vi "Parse GSA Sentence.vi"(8 "error in (no error)":errorcluster, 11 "GSA sentence":string) -> (0 "error out":errorcluster, 3 "GSA data":T1 {"type of fix"."mode" items=["", "No Fix", "2D Fix", "3D Fix"]; "selection of fix"."selection of 2D or 3D fix" items=["Automatic", "Manual"]})   [LabVIEW 2017, in "NMEA API.lvlib"]
doc: "Returns data contained in a particular type of NMEA sentence. The input sentence you specify must include valid NMEA formatting and end with a carriage return and line feed, or \\r\\n. You must manually select the polymorphic instance to use."
uses:
  <vilib>/robotics/Protocols/NMEA/NMEA API.lvlib
  <vilib>/robotics/Protocols/NMEA/typedefs/GSA Data.ctl
  <vilib>/robotics/Utilities/NI_Robotics Utilities.lvlib
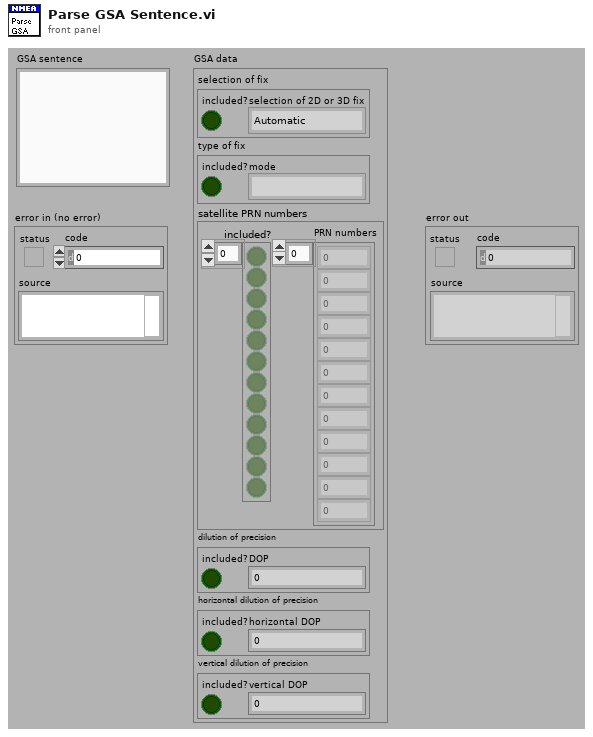
[diagram p1: front panel]
types:
  T1 = typedef "NMEA API.lvlib/GSA Data.ctl" = cluster{"selection of fix":cluster{"included?":bool, "selection of 2D or 3D fix":u16}, "type of fix":cluster{"included?":bool, "mode":u16}, "satellite PRN numbers":cluster{"included?":bool[], "PRN numbers":i32[]}, "dilution of precision":cluster{"included?":bool, "DOP":dbl}, "horizontal dilution of precision":cluster{"included?":bool, "horizontal DOP":dbl}, "vertical dilution of precision":cluster{"included?":bool, "vertical DOP":dbl}}
  T2 = cluster{"Included?":bool[], "Satellite PRNs":i32[]}
  T3 = cluster{"Valid?":bool, "Selection of 2D or 3D Fix":u16}
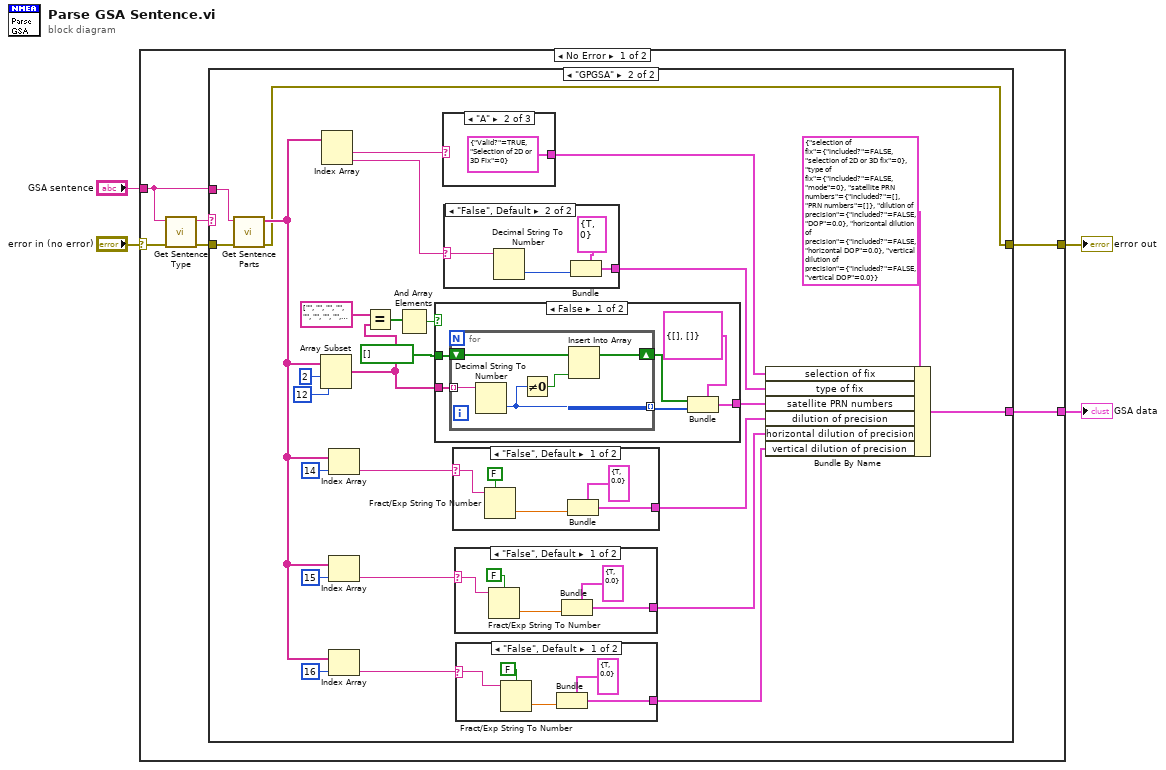
[diagram p0: block diagram]
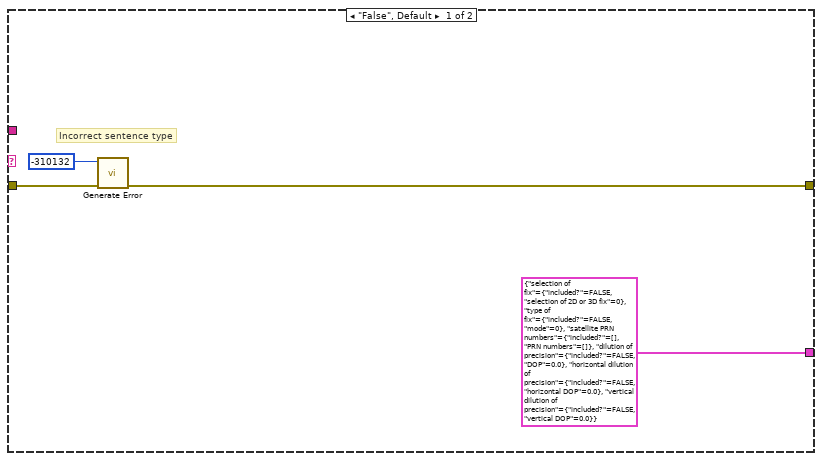
[diagram p2: hidden frame]
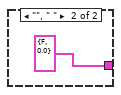
[diagram p3: hidden frame]
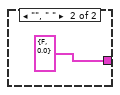
[diagram p4: hidden frame]
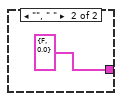
[diagram p5: hidden frame]
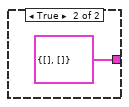
[diagram p6: hidden frame]
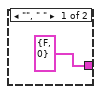
[diagram p7: hidden frame]
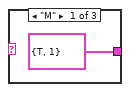
[diagram p8: hidden frame]
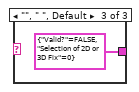
[diagram p9: hidden frame]
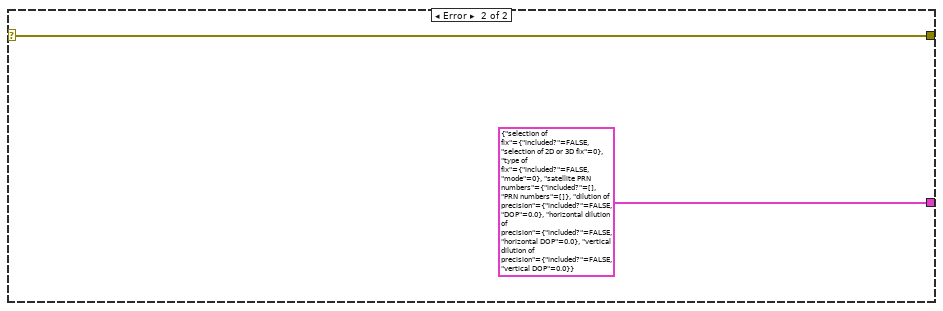
[diagram p10: hidden frame]
diagram:
  n1 = case shown="No Error" "error in (no error)" {
    selector: "error in (no error)" -> [w8 w81]
    tunnel: [w9 w81] -> w2
    tunnel: [w10 T1 {"selection of fix"={"included?"=FALSE, "selection of 2D or 3D fix"=0}, "type of fix"={"included?"=FALSE, "mode"=0}, "satellite PRN numbers"={"included?"=[], "PRN numbers"=[]}, "dilution of precision"={"included?"=FALSE, "DOP"=0.0}, "horizontal dilution of precision"={"included?"=FALSE, "horizontal DOP"=0.0}, "vertical dilution of precision"={"included?"=FALSE, "vertical DOP"=0.0}} ("GSA Data")] -> w1
    tunnel: "GSA sentence" -> [w6 _]
    frame No Error {
      n2 = call <vilib>:"Get Sentence Type.vi"("error in (no error)"=w8, "sentence"=w6) -> ("error out"=w7:errorcluster, "sentence type"=w5:string)  [unwired: 1 in, 7 out]
      n3 = case shown="\"GPGSA\"" w5 {
        tunnel: w6 -> [_ w16]
        tunnel: w7 -> [w12 w41]
        tunnel: [T1 {"selection of fix"={"included?"=FALSE, "selection of 2D or 3D fix"=0}, "type of fix"={"included?"=FALSE, "mode"=0}, "satellite PRN numbers"={"included?"=[], "PRN numbers"=[]}, "dilution of precision"={"included?"=FALSE, "DOP"=0.0}, "horizontal dilution of precision"={"included?"=FALSE, "horizontal DOP"=0.0}, "vertical dilution of precision"={"included?"=FALSE, "vertical DOP"=0.0}} ("GSA Data") w20] -> w10
        tunnel: [w11 w15] -> w9
        frame "False", Default {
          # "Incorrect sentence type"
          n4 = call <vilib>:"Generate Error.vi"("error in (no error)"=w12, "code"=-310132) -> ("error out"=w11:errorcluster)  [unwired: 9 in]
        }
        frame "GPGSA" {
          n5 = call <vilib>:"Get Sentence Parts.vi"("error in (no error)"=w41, "sentence"=w16) -> ("error out"=w15:errorcluster, "sentence data"=w17:string[])  [unwired: 1 in, 7 out]
          n6 = Array Subset(array=w17, index=2, length=12) -> (w32:string[])
          n7 = Index Array(array=w17) -> (element #1=w40:string, element #2=w36:string)  [unwired: 2 in]
          n8 = Index Array(array=w17, index=14) -> (element=w27:string)
          n9 = Index Array(array=w17, index=15) -> (element=w25:string)
          n10 = Index Array(array=w17, index=16) -> (element=w23:string)
          n11 = Equal?(x=string[] ["", "", "", "", "", "", "", "", "", "", "", ""], y=w32) -> (x = y?=w30:bool[])
          n12 = And Array Elements(Boolean array=w30) -> (logical AND=w29:bool)
          n13 = case shown="False" w29 {
            tunnel: w32 -> [w65 _]
            tunnel: [w62 T2 {"Included?"=[], "Satellite PRNs"=[]} ("Satellite PRNs")] -> w19
            tunnel: bool[] [] ("Included?") -> [w61 _]
            frame False {
              n14 = for {
                tunnel: [w66] -> w64 mode=indexing
                tunnel: w65 -> [w70] mode=indexing
                shift-right: [w68] -> w60
                shift-left: w61 -> [w69]
                n15 = Decimal String To Number(string=w70) -> (number=w66:i32)  [unwired: 3 out]
                n16 = Not Equal To 0?(x=w66) -> (x != 0?=w67:bool)
                n17 = Insert Into Array(array=w69, new element=w67) -> (w68:bool[])  [unwired: 1 in]
              }
              n18 = Bundle(cluster=T2 {"Included?"=[], "Satellite PRNs"=[]} ("Satellite PRNs"), "Included?"=w60, "Satellite PRNs"=w64) -> (w62:T2)
            }
            frame True {
            }
          }
          n19 = case shown="\"A\"" w40 {
            tunnel: [T3 {"Valid?"=TRUE, "Selection of 2D or 3D Fix"=1} ("Selection of Fix") T3 {"Valid?"=TRUE, "Selection of 2D or 3D Fix"=0} ("Selection of Fix") T3 {"Valid?"=FALSE, "Selection of 2D or 3D Fix"=0} ("Selection of Fix")] -> w35
            frame "M" {
            }
            frame "A" {
            }
            frame "", " ", Default {
            }
          }
          n20 = case shown="\"False\", Default" w36 {
            selector: w36 -> [_ w76]
            tunnel: [cluster{"Valid?":bool, "Type of Fix":u16} {"Valid?"=FALSE, "Type of Fix"=0} ("Type of Fix") w73] -> w28
            frame "", " " {
            }
            frame "False", Default {
              n21 = Decimal String To Number(string=w76) -> (number=w74:i32)  [unwired: 3 out]
              n22 = Bundle(cluster=cluster{"Valid?":bool, "Type of Fix":u16} {"Valid?"=TRUE, "Type of Fix"=0} ("Type of Fix"), "Type of Fix"=w74) -> (w73:cluster{"Valid?":bool, "Type of Fix":u16})  [unwired: 1 out]
            }
          }
          n23 = case shown="\"False\", Default" w27 {
            selector: w27 -> [w58 _]
            tunnel: [w55 cluster{"Valid?":bool, "DOP":dbl} {"Valid?"=FALSE, "DOP"=0.0} ("Dilution of Precision")] -> w26
            frame "False", Default {
              n24 = Fract/Exp String To Number(use system decimal point (T)=FALSE, string=w58) -> (number=w56:dbl)  [unwired: 3 out]
              n25 = Bundle(cluster=cluster{"Valid?":bool, "DOP":dbl} {"Valid?"=TRUE, "DOP"=0.0} ("Dilution of Precision"), "DOP"=w56) -> (w55:cluster{"Valid?":bool, "DOP":dbl})  [unwired: 1 out]
            }
            frame "", " " {
            }
          }
          n26 = case shown="\"False\", Default" w25 {
            selector: w25 -> [w52 _]
            tunnel: [w49 cluster{"Valid?":bool, "DOP":dbl} {"Valid?"=FALSE, "DOP"=0.0} ("Dilution of Precision")] -> w24
            frame "False", Default {
              n27 = Fract/Exp String To Number(use system decimal point (T)=FALSE, string=w52) -> (number=w50:dbl)  [unwired: 3 out]
              n28 = Bundle(cluster=cluster{"Valid?":bool, "DOP":dbl} {"Valid?"=TRUE, "DOP"=0.0} ("Dilution of Precision"), "DOP"=w50) -> (w49:cluster{"Valid?":bool, "DOP":dbl})  [unwired: 1 out]
            }
            frame "", " " {
            }
          }
          n29 = case shown="\"False\", Default" w23 {
            selector: w23 -> [w46 _]
            tunnel: [w43 cluster{"Valid?":bool, "DOP":dbl} {"Valid?"=FALSE, "DOP"=0.0} ("Dilution of Precision")] -> w22
            frame "False", Default {
              n30 = Fract/Exp String To Number(use system decimal point (T)=FALSE, string=w46) -> (number=w44:dbl)  [unwired: 3 out]
              n31 = Bundle(cluster=cluster{"Valid?":bool, "DOP":dbl} {"Valid?"=TRUE, "DOP"=0.0} ("Dilution of Precision"), "DOP"=w44) -> (w43:cluster{"Valid?":bool, "DOP":dbl})  [unwired: 1 out]
            }
            frame "", " " {
            }
          }
          n32 = Bundle By Name(cluster=T1 {"selection of fix"={"included?"=FALSE, "selection of 2D or 3D fix"=0}, "type of fix"={"included?"=FALSE, "mode"=0}, "satellite PRN numbers"={"included?"=[], "PRN numbers"=[]}, "dilution of precision"={"included?"=FALSE, "DOP"=0.0}, "horizontal dilution of precision"={"included?"=FALSE, "horizontal DOP"=0.0}, "vertical dilution of precision"={"included?"=FALSE, "vertical DOP"=0.0}} ("GSA Data"), "selection of fix"=w35, "type of fix"=w28, "satellite PRN numbers"=w19, "dilution of precision"=w26, "horizontal dilution of precision"=w24, "vertical dilution of precision"=w22) -> (w20:T1)
        }
      }
    }
    frame Error {
    }
  }
  "error out" <- w2
  "GSA data" <- w1
